vi "read_T1.vi"(11 "file_path":path) -> (0 "fitted_signal":T2, 1 "fit_parameters":T4 {"mse" format="%.3g"; "T1" format="%.3g"; "C1" format="%.3g"; "Tm" format="%.3g"; "Cm" format="%.3g"; "Ie" format="%.3g"}, 2 "T1_curve":T3, 3 "T1_parameters":T1, 4 "file_path":path, 5 "timetags":u32[][](array[numeric]), 7 "triggers":u32[][](array[numeric]))   [LabVIEW 2014]
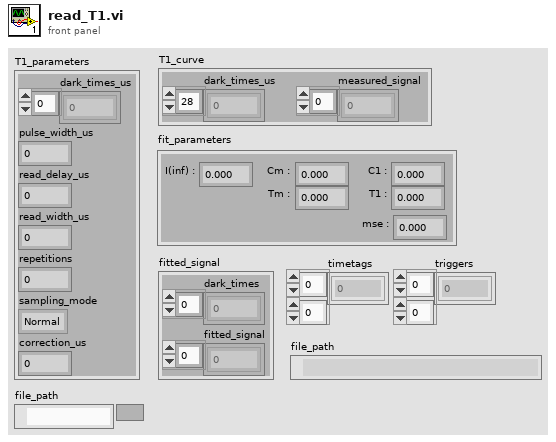
[diagram p1: front panel]
types:
  T1 = cluster{"dark_times_us":dbl[], "pulse_width_us":dbl, "read_delay_us":dbl, "read_width_us":dbl, "repetitions":i32, "sampling_mode":enum16{"Normal", "Sweep"}, "correction_us":dbl}
  T2 = cluster{"dark_times":dbl[], "fitted_signal":dbl[]}
  T3 = cluster{"dark_times_us":dbl[], "measured_signal":dbl[]}
  T4 = cluster{"Ie":dbl, "Cm":dbl, "Tm":dbl, "C1":dbl, "T1":dbl, "mse":dbl}
  T5 = enum16{"open", "replace", "create", "open or create", "replace or create", "replace or create with confirmation"}
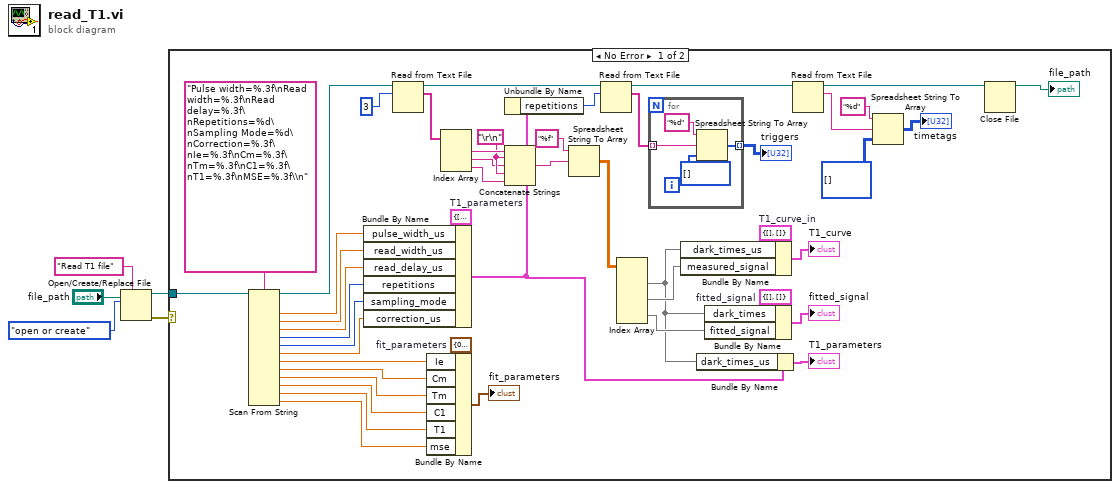
[diagram p0: block diagram]
diagram:
  n1 = Open/Create/Replace File(file path (use dialog)="file_path", prompt="Read T1 file", operation (0:open)=T5."open or create") -> (refnum out=w2:refnum<file>, error out=w3:errorcluster)  [unwired: 3 in, 1 out]
  n2 = case shown="No Error" w3 {
    tunnel: w2 -> [w14 _]
    frame No Error {
      w19 = T1 {"dark_times_us"=[], "pulse_width_us"=0.0, "read_delay_us"=0.0, "read_width_us"=0.0, "repetitions"=0, "sampling_mode"=enum."Normal", "correction_us"=0.0}  # T1_parameters
      w22 = "\r\n"
      w36 = T3 {"dark_times_us"=[], "measured_signal"=[]}  # T1_curve_in
      w37 = T2 {"dark_times"=[], "fitted_signal"=[]}  # fitted_signal
      w47 = T4 {"Ie"=0.0, "Cm"=0.0, "Tm"=0.0, "C1"=0.0, "T1"=0.0, "mse"=0.0}  # fit_parameters
      n3 = Scan From String("Pulse width=%.3f\nRead width=%.3f\nRead delay=%.3f\nRepetitions=%d\nSampling Mode=%d\nCorrection=%.3f\nIe=%.3f\nCm=%.3f\nTm=%.3f\nC1=%.3f\nT1=%.3f\nMSE=%.3f\\n" ("format string"), w14) -> (w39:refnum<file>, output 1=w49:dbl, output 2=w50:dbl, output 3=w51:dbl, output 4=w52:i32, output 5=w18:i32, output 6=w17:dbl, output 7=w45:dbl, output 8=w44:dbl, output 9=w43:dbl, output 10=w42:dbl, output 11=w41:dbl, output 12=w40:dbl)  [unwired: 13 in, 1 out]
      n4 = Bundle By Name(cluster=w19, "pulse_width_us"=w49, "read_width_us"=w50, "read_delay_us"=w51, "repetitions"=w52, "sampling_mode"=w18, "correction_us"=w17) -> (w9:T1)
      n5 = Read from Text File(file (use dialog)=w39, count=3) -> (refnum out=w11:refnum<file>, text=w28:string[])  [unwired: 2 in, 2 out]
      n6 = Bundle By Name(cluster=w47, "Ie"=w45, "Cm"=w44, "Tm"=w43, "C1"=w42, "T1"=w41, "mse"=w40) -> (→"fit_parameters":T4)
      n7 = Index Array(array=w28) -> (element #1=w30:string, element #2=w21:string, element #3=w20:string)  [unwired: 3 in]
      n8 = Unbundle By Name(w9) -> ("repetitions"=w8:i32)
      n9 = Concatenate Strings(w30, w22, w21, w22, w20) -> (w27:string)
      n10 = Spreadsheet String To Array(format string="%f", spreadsheet string=w27) -> (array=w33:dbl[][])  [unwired: 2 in]
      n11 = Read from Text File(file (use dialog)=w11, count=w8) -> (refnum out=w10:refnum<file>, text=w7:string[])  [unwired: 2 in, 2 out]
      n12 = Index Array(array=w33) -> (element #1=w15:dbl[], element #2=w32:dbl[], element #3=w31:dbl[])  [unwired: 6 in]
      n13 = for {
        tunnel: w7 -> [w54] mode=indexing
        tunnel: [w53] -> w6 mode=indexing
        n14 = Spreadsheet String To Array(format string="%d", spreadsheet string=w54, array type (2D Dbl)=u32[] [] ("triggers")) -> (array=w53:u32[])  [unwired: 1 in]
      }
      "triggers" <- w6
      n15 = Bundle By Name(cluster=w36, "dark_times_us"=w15, "measured_signal"=w32) -> (→"T1_curve":T3)
      n16 = Bundle By Name(cluster=w9, "dark_times_us"=w15) -> (→"T1_parameters":T1)
      n17 = Bundle By Name(cluster=w37, "dark_times"=w15, "fitted_signal"=w31) -> (→"fitted_signal":T2)
      n18 = Read from Text File(file (use dialog)=w10) -> (refnum out=w13:refnum<file>, text=w25:string)  [unwired: 3 in, 2 out]
      n19 = Spreadsheet String To Array(format string="%d", spreadsheet string=w25, array type (2D Dbl)=u32[][] []) -> (array=→"timetags":u32[][])  [unwired: 1 in]
      n20 = Close File(refnum=w13) -> (path=→"file_path":path)  [unwired: 1 in, 1 out]
    }
    frame Error {
    }
  }
